vi "Initialize.vi"(7 "Serial Configuration":T1={"Baud Rate"=9600, "Parity"=0, "Data Bits"=8, "Stop Bits"=10, "Flow Control"=0} {"Flow Control" items=["None", "XON/XOFF", "RTS/CTS", "XON/XOFF & RTS/CTS", "DTR/DSR", "XON/XOFF & DTR/DSR"]; "Stop Bits" items=["1.0"=10, "1.5"=15, "2.0"=20]; "Data Bits" items=["7"=7, "8"=8]; "Parity" items=["None", "Odd", "Even", "Mark", "Space"]; "Baud Rate" items=["300"=300, "600"=600, "1200"=1200, "2400"=2400, "4800"=4800, "9600"=9600, "19200"=19200]}, 8 "error in (no error)":errorcluster, 9 "Address (0)":i32, 10 "ID Query (True)":bool=TRUE, 11 "VISA resource name":refnum<visa-resource-name>) -> (0 "error out":errorcluster, 3 "VISA resource name out":refnum<visa-resource-name>)   [LabVIEW 2016, in "Environment Chamber.lvlib" / "Climatic Chamber.lvlib"]
doc: "Establishes communication with the instrument and optionally performs an instrument identification query.\nTherefore, call this VI before calling other instrument driver VIs for this instrument.\nGenerally, you need to call the Initialize VI only once at the beginning of an application.\n\n<b>RS-232 / RS-485 Communication</b>"
uses:
  Climatic Chamber.lvlib
panel:
  # "(c) 2015 <Espec Corp.>.  ALL RIGHTS RESERVED."
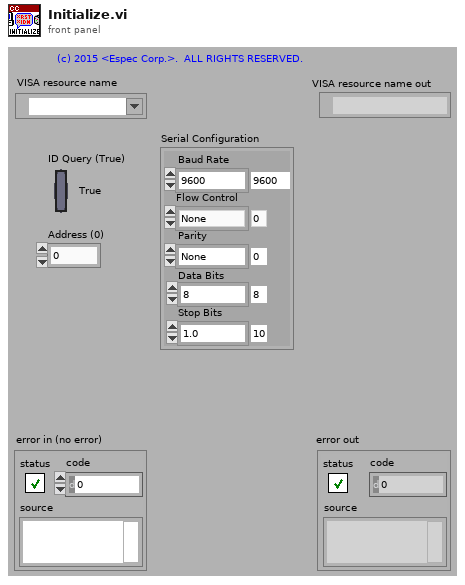
[diagram p1: front panel]
types:
  T1 = cluster{"Baud Rate":u32, "Parity":u16, "Data Bits":u16, "Stop Bits":u16, "Flow Control":u16}
  T2 = typedef "Environment Chamber.lvlib/Climatic Chamber.lvlib/Chamber Type Cluster.ctl" = cluster{"dry bulb sensor":T3, "Temp. only chamber":bool, "wet bulb sensor":T3, "Controller type":string, "Temp. upper limit":dbl}
  T3 = typedef "Environment Chamber.lvlib/Climatic Chamber.lvlib/Sensor Type Enum.ctl" = enum16{"Not defined", "Thermocouple"}
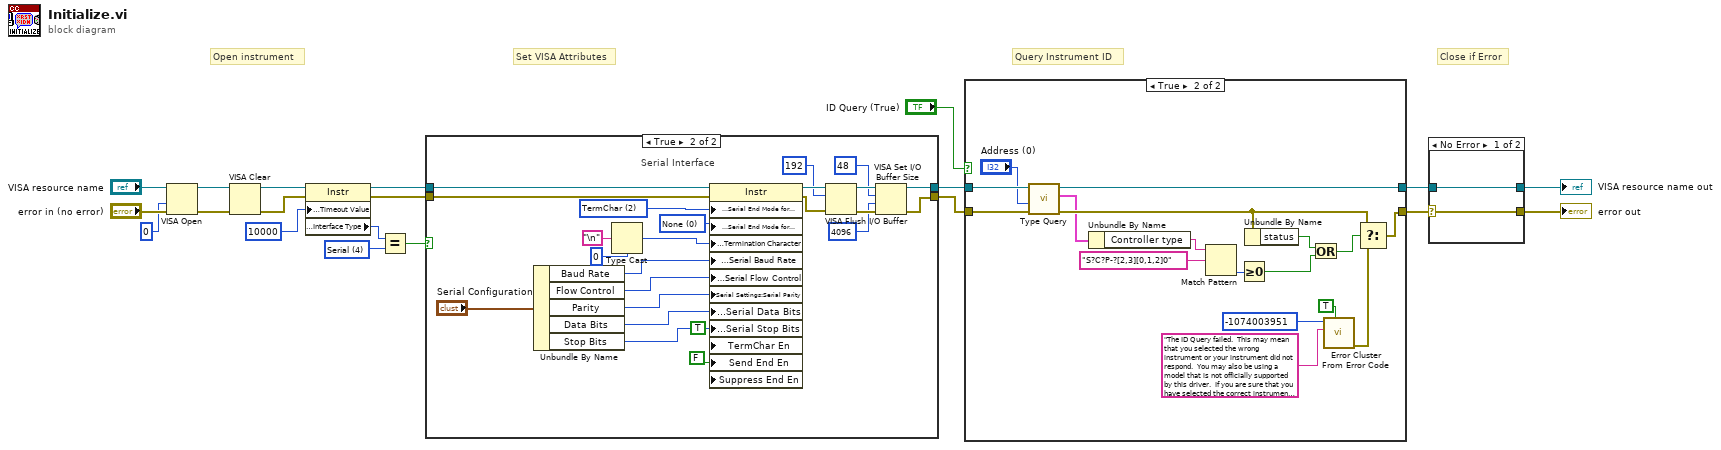
[diagram p0: block diagram]
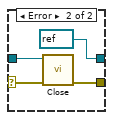
[diagram p3: hidden frame]
diagram:
  w10 = u16 4 items=["GPIB"=1, "VXI"=2, "GPIB-VXI"=3, "Serial"=4, "PXI"=5, "TCPIP"=6, "USB"=7] ("Interface Information:Interface Type")
  # "Set VISA Attributes"
  # "Close if Error"
  # "Query Instrument ID"
  # "Open instrument"
  n1 = VISA Open(access mode=u32 0, error in (no error)="error in (no error)", VISA resource name="VISA resource name") -> (VISA resource name=w8:refnum<visa-resource-name>, error out=w7:errorcluster)  [unwired: 2 in]
  n2 = VISA Clear(VISA resource name=w8, error in (no error)=w7) -> (VISA resource name out=w6:refnum<visa-resource-name>, error out=w5:errorcluster)
  n3 = property class="Instr"(reference=w6, error in=w5, "General Settings:Timeout Value"=u32 10000) -> (reference out=w13:refnum<visa-resource-name>, error out=w12:errorcluster, "Interface Information:Interface Type"=w17:u16)
  n4 = Equal?(x=w17, y=w10) -> (x = y?=w11:bool)
  n5 = case shown="True" w11 {
    tunnel: [w21 w43] -> w15
    tunnel: [w22 w40] -> w14
    tunnel: w13 -> [w21 w45]
    tunnel: w12 -> [w22 w46]
    frame False {
      # "EDIT: Remove interfaces not\nsupported by your instrument."
      # "GPIB, TCP/IP, and USB Interface"
    }
    frame True {
      w23 = u16 0 items=["None", "Last Bit", "TermChar", "Break"] ("Serial Settings:End Mode for Writes")
      w24 = FALSE ("Message Based Settings:Suppress End Enable")
      w33 = u16 2 items=["None", "LastBit", "TermChar"] ("Serial Settings:Serial End Mode for Reads")
      # "Serial Interface"
      n6 = Unbundle By Name("Serial Configuration") -> ("Baud Rate"=w31:u32, "Flow Control"=w27:u16, "Parity"=w29:u16, "Data Bits"=w30:u16, "Stop Bits"=w26:u16)
      n7 = Type Cast(type=u8 0, x="\n" ("Line Feed Constant")) -> (*(type *) &x=w32:u8)
      n8 = property class="Instr"(reference=w45, error in=w46, "Serial Settings:Serial End Mode for Reads"=w33, "Serial Settings:Serial End Mode for Writes"=w23, "Message Based Settings:Termination Character"=w32, "Serial Settings:Serial Baud Rate"=w31, "Serial Settings:Serial Flow Control"=w27, "Serial Settings:Serial Parity"=w29, "Serial Settings:Serial Data Bits"=w30, "Serial Settings:Serial Stop Bits"=w26, "TermChar En"=TRUE ("Message Based Settings:Send End Enable"), "Send End En"=w24, "Suppress End En"=w24) -> (reference out=w39:refnum<visa-resource-name>, error out=w42:errorcluster)
      n9 = VISA Flush I/O Buffer(VISA resource name=w39, mask (16)=u16 192, error in (no error)=w42) -> (VISA resource name out=w44:refnum<visa-resource-name>, error out=w41:errorcluster)
      n10 = VISA Set I/O Buffer Size(VISA resource name=w44, mask (16)=u16 48, size (4096)=u32 4096 ("size (0)"), error in (no error)=w41) -> (VISA resource name out=w43:refnum<visa-resource-name>, error out=w40:errorcluster)
    }
  }
  n11 = case shown="True" "ID Query (True)" {
    tunnel: [w47 w65] -> w1
    tunnel: [w48 w53] -> w2
    tunnel: w15 -> [w48 w55]
    tunnel: w14 -> [w47 w54]
    frame False {
    }
    frame True {
      n12 = call "Type Query.vi"("error in (no error)"=w54, "Address (0)"="Address (0)", "VISA resource name"=w55) -> ("error out"=w52:errorcluster, "Chamber Type"=w50:T2, "VISA resource name out"=w53:refnum<visa-resource-name>)  [unwired: 6 in]
      n13 = Unbundle By Name(w50) -> ("Controller type"=w49:string)
      n14 = Match Pattern(string=w49, regular expression="S?C?P-?[2,3][0,1,2]0") -> (offset past match=w59:i32)  [unwired: 1 in, 3 out]
      n15 = Greater Or Equal To 0?(x=w59) -> (x >= 0?=w57:bool)
      n16 = Unbundle By Name(w52) -> ("status"=w58:bool)
      n17 = Or(x=w58, y=w57) -> (x .or. y?=w56:bool)
      n18 = call <vilib>:"Error Cluster From Error Code.vi"("show call chain? (False)"=TRUE, "error message (\"\")"="The ID Query failed.  This may mean that you selected the wrong instrument or your instrument did not respond.  You may also be using a model that is not officially supported by this driver.  If you are sure that you have selected the correct instrument and it is responding, try disabling the ID Query." ("Source (VI Name)"), "error code (0)"=-1074003951 ("Code")) -> ("error out"=w63:errorcluster)  [unwired: 6 in]
      n19 = Select(t=w52, s=w56, f=w63) -> (s? t:f=w65:errorcluster)
    }
  }
  n20 = case shown="No Error" w1 {
    selector: w1 -> [w66 w69]
    tunnel: w2 -> [w67 w70]
    tunnel: [w67 refnum<visa-resource-name> refnum ("VISA resource name out")] -> w4
    tunnel: [w66 w71] -> w3
    frame No Error {
    }
    frame Error {
      n21 = call "Close.vi"("error in (no error)"=w69, "VISA resource name"=w70) -> ("error out"=w71:errorcluster)  [unwired: 9 in]
    }
  }
  "VISA resource name out" <- w4
  "error out" <- w3
